vi "Reference.vi"(0 "AI Config":T2={"AI Rate"=200000.0, "AI Block Size"=40000, "AI Buffer Size (s)"=10, "AI.Coupling"=10050, "AI.Max"=10.0, "AI.Min"=-10.0, "Input physical channels"="PXI1Slot3/ai0:1"}, 1 "Reset":bool, 2 "Ref Amp":dbl=5.0 format="%.2f", 3 "Ref Shape":enum16{"Sine", "Square"}(ring), 4 "Phase&time":T1, 5 "Frequency":dbl=20.0 format="%.2f", 7 "Phase log in":dbl=0.9999999999996251) -> (6 "Phase log":dbl=0.9999999999996251, 8 "Ref out":T3={"Ref X"=array[40000 elements], "Ref Y"=array[40000 elements], "AI Rate"=200000.0, "AI Block Size"=40000.0, "Frequency"=20.0, "Ref amp"=5.0} {"Ref amp" step=0.001 format="%0.4f"; "Frequency" step=0.001 format="%0.4f"; "AI Block Size" step=0.001 format="%0.4f"; "AI Rate" step=0.001 format="%0.4f"})   [LabVIEW 2011]
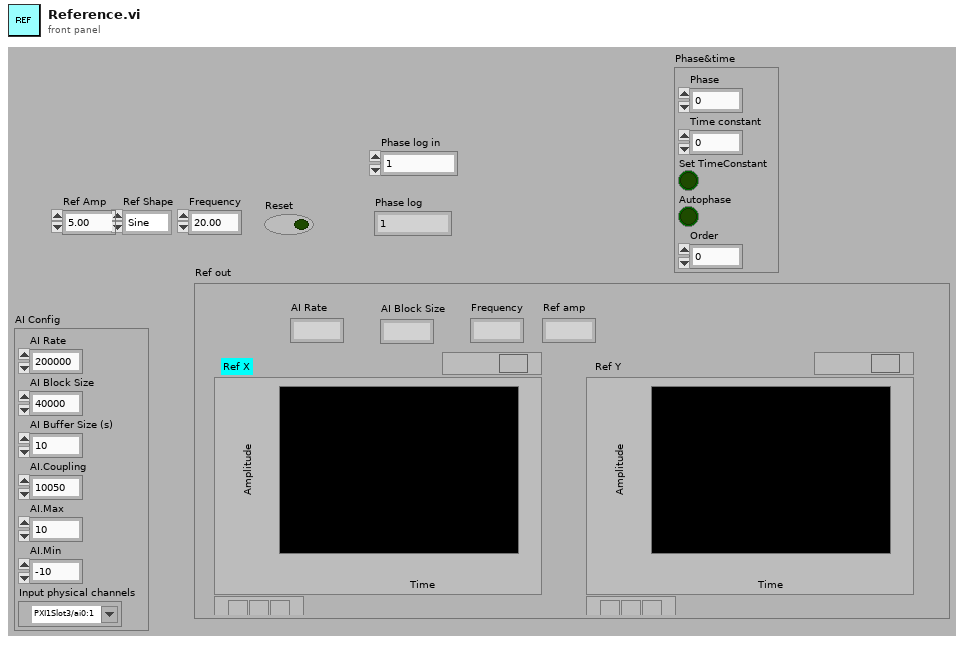
[diagram p1: front panel]
types:
  T1 = cluster{"Phase":dbl, "Time constant":dbl, "Set TimeConstant":bool, "Autophase":bool, "Order":dbl}
  T2 = cluster{"AI Rate":dbl, "AI Block Size":i32, "AI Buffer Size (s)":i32, "AI.Coupling":i32, "AI.Max":dbl, "AI.Min":dbl, "Input physical channels":tag}
  T3 = cluster{"Ref X":dbl[], "Ref Y":dbl[], "AI Rate":dbl, "AI Block Size":dbl, "Frequency":dbl, "Ref amp":dbl}
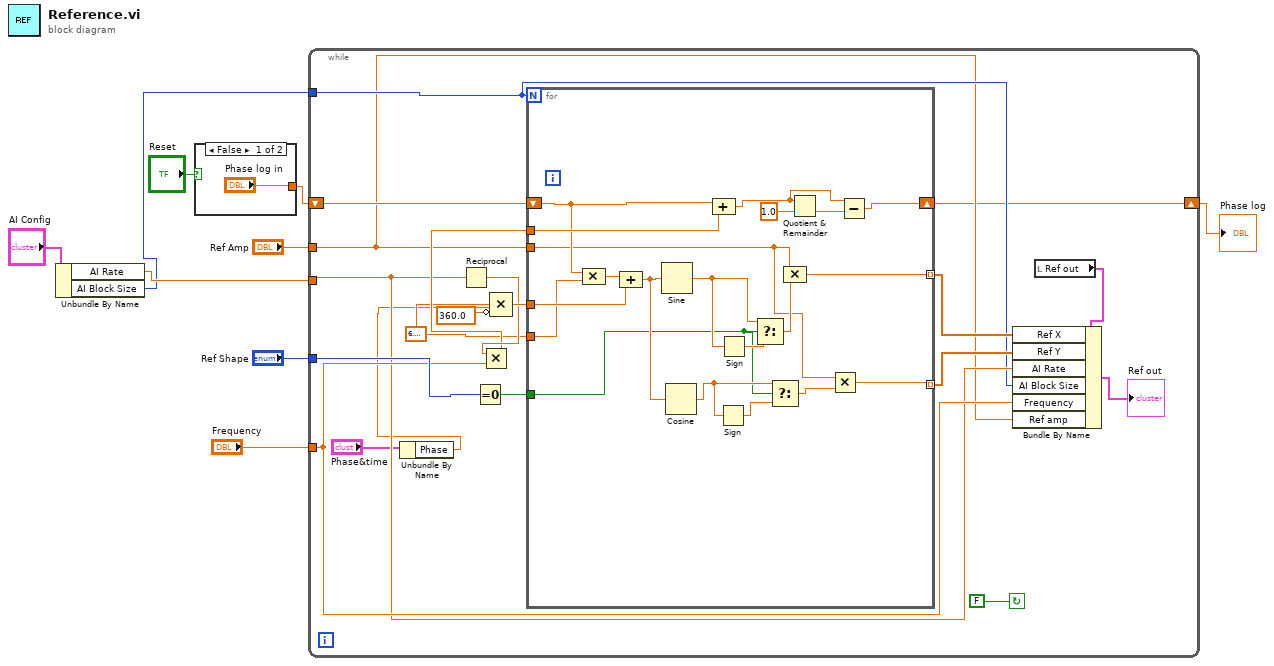
[diagram p0: block diagram]
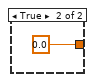
[diagram p2: hidden frame]
diagram:
  n1 = Unbundle By Name("AI Config") -> ("AI Rate"=w3:dbl, "AI Block Size"=w2:i32)
  n2 = case shown="False" "Reset" {
    tunnel: ["Phase log in" 0.0] -> w6
    frame False {
    }
    frame True {
    }
  }
  n3 = while {
    shift-left: w6 -> [w31]
    shift-right: [w12] -> w1
    tunnel: w2 -> [w18]
    tunnel: "Ref Amp" -> [w17]
    tunnel: w3 -> [w19]
    tunnel: "Ref Shape" -> [w26]
    tunnel: "Frequency" -> [w20]
    stop <- FALSE continue-if-true
    w23 = 6.283185307179586
    n4 = Unbundle By Name("Phase&time") -> ("Phase"=w13:dbl)
    n5 = Reciprocal(x=w19) -> (1/x=w25:dbl)
    n6 = Equal To 0?(x=w26) -> (x = 0?=w29:bool)
    n7 = Multiply(x=w25, y=w20) -> (x*y=w24:dbl)
    n8 = Compound Arithmetic op=MULTIPLY(w13, w23, invert 360.0 ("value")) -> (w28:dbl)
    n9 = for {
      N: w18 -> [_]
      shift-right: [w40] -> w12
      shift-left: w31 -> [w45]
      tunnel: w24 -> [w51]
      tunnel: w17 -> [w33]
      tunnel: w29 -> [w35]
      tunnel: w28 -> [w48]
      tunnel: [w44] -> w22 mode=indexing
      tunnel: w23 -> [w39]
      tunnel: [w32] -> w21 mode=indexing
      n10 = Compound Arithmetic op=MULTIPLY(w45, w39) -> (w49:dbl)
      n11 = Compound Arithmetic op=ADD(w49, w48) -> (w38:dbl)
      n12 = Sine(x=w38) -> (sin(x)=w47:dbl)
      n13 = Cosine(x=w38) -> (cos(x)=w37:dbl)
      n14 = Compound Arithmetic op=ADD(w45, w51) -> (w42:dbl)
      n15 = Sign(1:w37) -> (0:w36:dbl)
      n16 = Sign(1:w47) -> (0:w46:dbl)
      n17 = Select(t=w47, s=w35, f=w46) -> (s? t:f=w50:dbl)
      n18 = Select(t=w37, s=w35, f=w36) -> (s? t:f=w34:dbl)
      n19 = Compound Arithmetic op=MULTIPLY(w33, w50) -> (w44:dbl)
      n20 = Quotient & Remainder(x=w42, y=1.0) -> (floor(x/y)=w41:dbl)  [unwired: 1 out]
      n21 = Multiply(x=w33, y=w34) -> (x*y=w32:dbl)
      n22 = Subtract(x=w42, y=w41) -> (x-y=w40:dbl)
    }
    n23 = local read "Ref out"() -> (w16:T3)
    n24 = Bundle By Name(cluster=w16, "Ref X"=w22, "Ref Y"=w21, "AI Rate"=w19, "AI Block Size"=w18, "Frequency"=w20, "Ref amp"=w17) -> (→"Ref out":T3)
  }
  "Phase log" <- w1
